vi "Read Id.vi"(8 "error in (no error)":errorcluster, 11 "CommandDirector in":refnum<class "CommandDirector.lvclass">) -> (0 "error out":errorcluster, 2 "Id":string, 3 "CommandDirector out":refnum<class "CommandDirector.lvclass">)   [LabVIEW 2023, in "HAF.lvlib" / "CommandDirector.lvclass"]
doc: "Returns the Director's Id. If blank, sets a new one based on a generated UUID."
uses:
  CommandDirector.lvclass
  CommandDirector.lvclass/CommandDirector.ctl
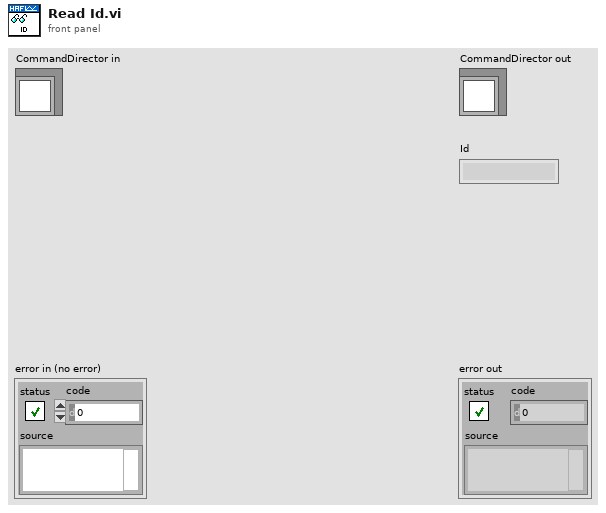
[diagram p1: front panel]
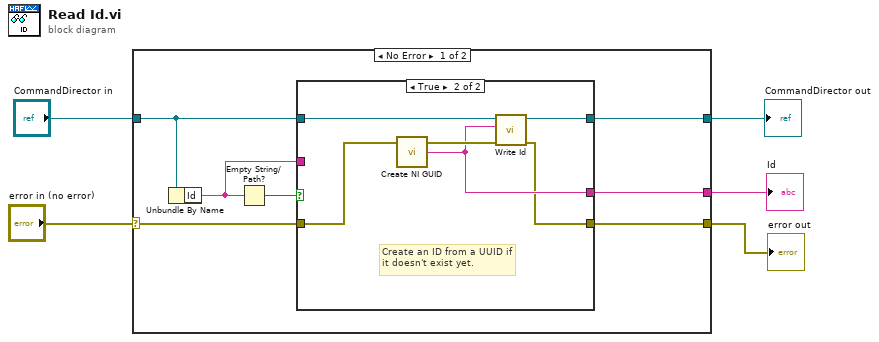
[diagram p0: block diagram]
diagram:
  n1 = case shown="No Error" "error in (no error)" {
    selector: "error in (no error)" -> [w10 w21]
    tunnel: [w6 w21] -> w4
    tunnel: [w8 w22] -> w2
    tunnel: "CommandDirector in" -> [w12 w22]
    tunnel: [w7 _] -> w1
    frame No Error {
      n2 = Unbundle By Name(w12) -> ("Id"=w9:string)
      n3 = Empty String/Path?(string/path=w9) -> (empty?=w11:bool)
      n4 = case shown="True" w11 {
        tunnel: w12 -> [w14 w20]
        tunnel: w10 -> [w13 w19]
        tunnel: w9 -> [w15 _]
        tunnel: [w14 w18] -> w8
        tunnel: [w15 w17] -> w7
        tunnel: [w13 w16] -> w6
        frame False {
        }
        frame True {
          # "Create an ID from a UUID if it doesn't exist yet."
          n5 = call <vilib>:"Create NI GUID.vi"() -> ("NI GUID"=w17:string)
          n6 = call-dynamic "Write Id.vi"("error in (no error)"=w19, "Id"=w17, "CommandDirector in"=w20) -> ("error out"=w16:errorcluster, "CommandDirector out"=w18:refnum<class "CommandDirector.lvclass">)  [unwired: 7 in]
        }
      }
    }
    frame Error {
    }
  }
  "error out" <- w4
  "CommandDirector out" <- w2
  "Id" <- w1
